vi "Sub_Pin_Location_to_Node.vi"(10 "Pin Location":dbl, 11 "Setup Parameters":T1) -> (3 "DOF of Interest":i32)   [LabVIEW 2019]
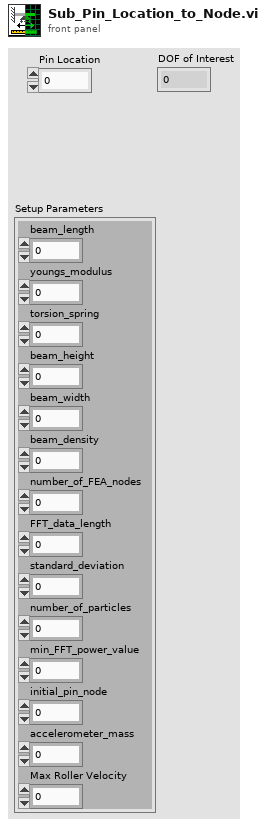
[diagram p1: front panel]
types:
  T1 = cluster{"beam_length":dbl, "youngs_modulus":dbl, "torsion_spring":dbl, "beam_height":dbl, "beam_width":dbl, "beam_density":dbl, "number_of_FEA_nodes":i32, "FFT_data_length":i32, "standard_deviation":dbl, "number_of_particles":i32, "min_FFT_power_value":dbl, "initial_pin_node":i32, "accelerometer_mass":dbl, "Max Roller Velocity":dbl}
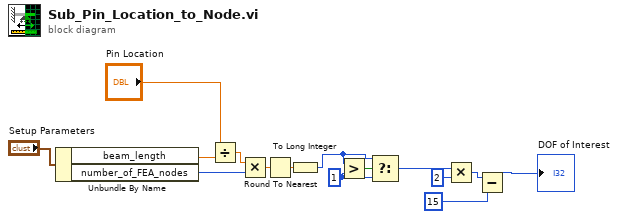
[diagram p0: block diagram]
diagram:
  w6 = 1 ("y")
  n1 = Unbundle By Name("Setup Parameters") -> ("beam_length"=w4:dbl, "number_of_FEA_nodes"=w3:i32)
  n2 = Divide(x="Pin Location", y=w4) -> (x/y=w12:dbl)
  n3 = Multiply(x=w12, y=w3) -> (x*y=w11:dbl)
  n4 = Round To Nearest(number=w11) -> (nearest integer value=w10:dbl)
  n5 = To Long Integer(number=w10) -> (32bit integer=w8:i32)
  n6 = Greater?(x=w8, y=w6) -> (0:w9:bool)
  n7 = Select(t=w8, s=w9, f=w6) -> (s? t:f=w7:i32)
  n8 = Multiply(x=w7, y=2) -> (x*y=w14:i32)
  n9 = Subtract(x=w14, y=15) -> (x-y=→"DOF of Interest":i32)
